vi "ArduinoMicro Module.vi"(5 "Enable":bool=TRUE, 6 "Timeout(s)":dbl=2.0, 7 "Command":T3, 8 "error in (no error)":errorcluster, 10 "VALVES":T1, 11 "VISA resource name":refnum<visa-resource-name>="COM39") -> (0 "error out":errorcluster, 1 "Output":T2, 2 "read string":string, 3 "TimeOut":bool, 4 "write string":string)   [LabVIEW 2017]
uses:
  ArduinoMicro Module Control.ctl
  KISSIA_VALVULAS.ctl
  <vilib>/Instr/_visa.llb/VISA Configure Serial Port (Instr).vi
panel:
  # "Input Data"
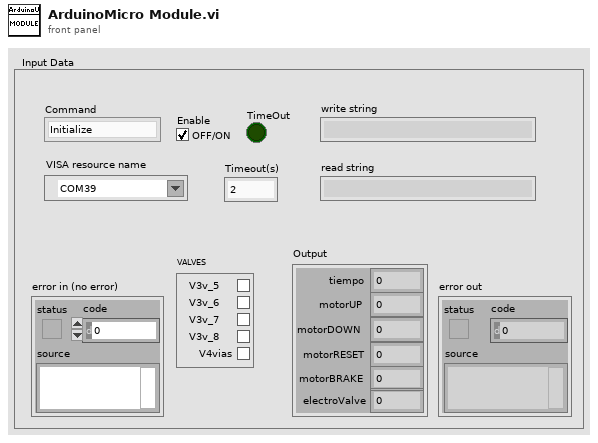
[diagram p1: front panel]
types:
  T1 = typedef "KISSIA_VALVULAS.ctl" = cluster{"V3v_5":bool, "V3v_6":bool, "V3v_7":bool, "V3v_8":bool, "V4vias":bool}
  T2 = cluster{"tiempo":dbl, "motorUP":dbl, "motorDOWN":dbl, "motorRESET":dbl, "motorBRAKE":dbl, "electroValve":dbl}
  T3 = typedef "ArduinoMicro Module Control.ctl" = enum16{"Initialize", "Read Data", "Write Data", "Enable", "Disable", "Shutdown"}
  T4 = cluster{"tiempo":dbl, "Valvula":dbl, "motorUP":dbl, "motorDOWN":dbl, "motorRESET":dbl, "motorBRAKE":dbl}
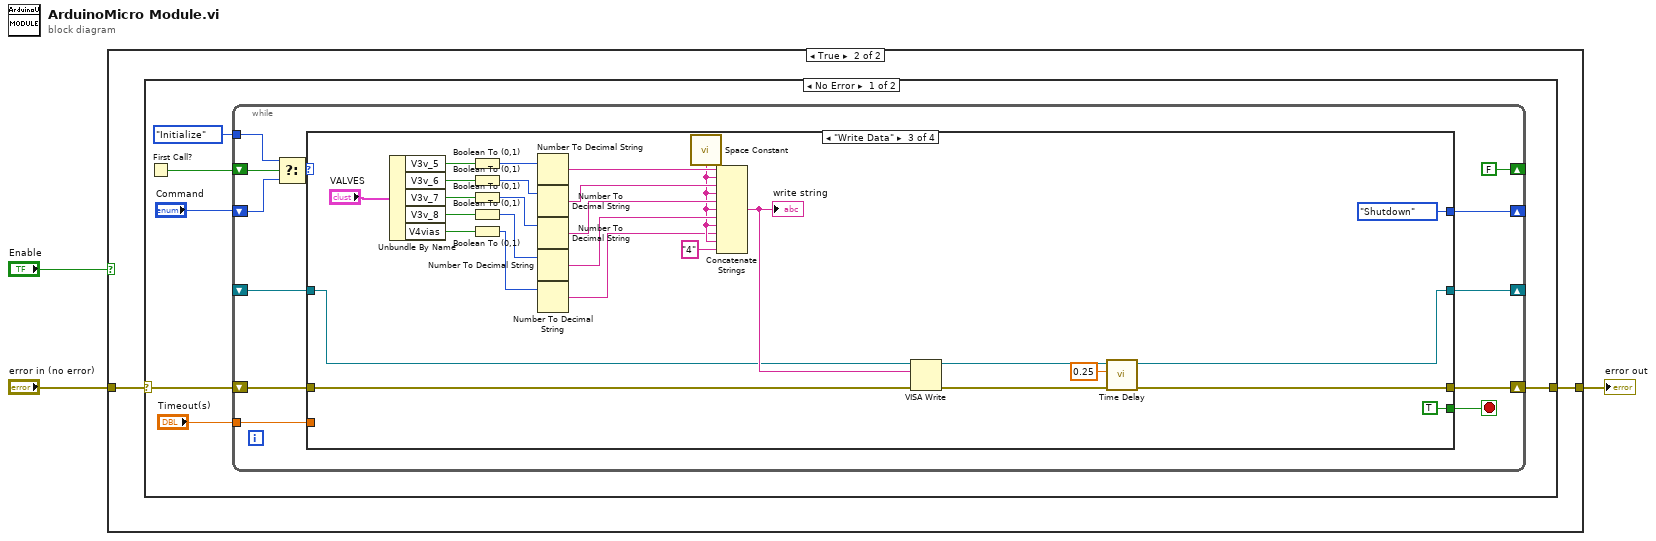
[diagram p0: block diagram]
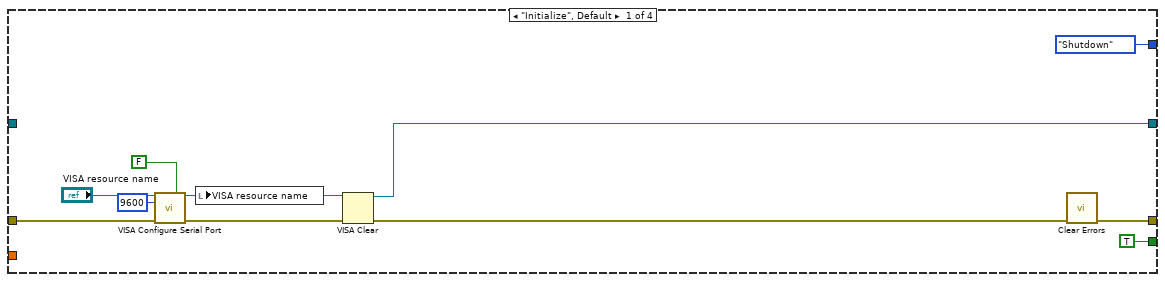
[diagram p3: hidden frame]
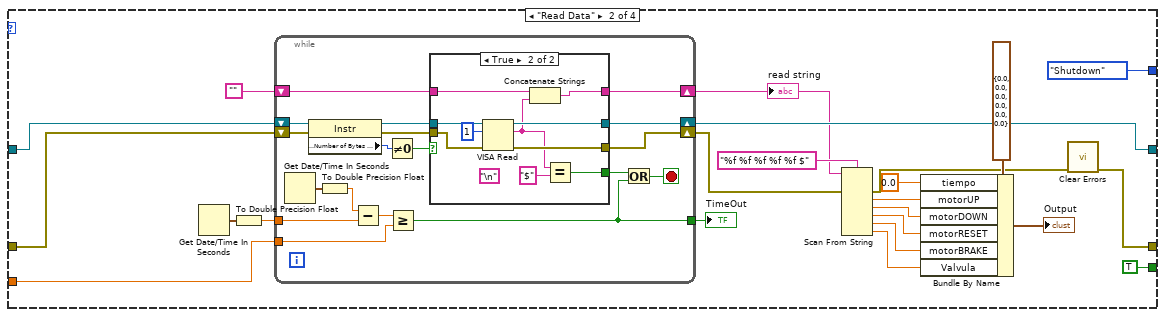
[diagram p4: hidden frame]
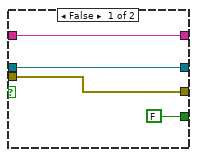
[diagram p5: hidden frame]
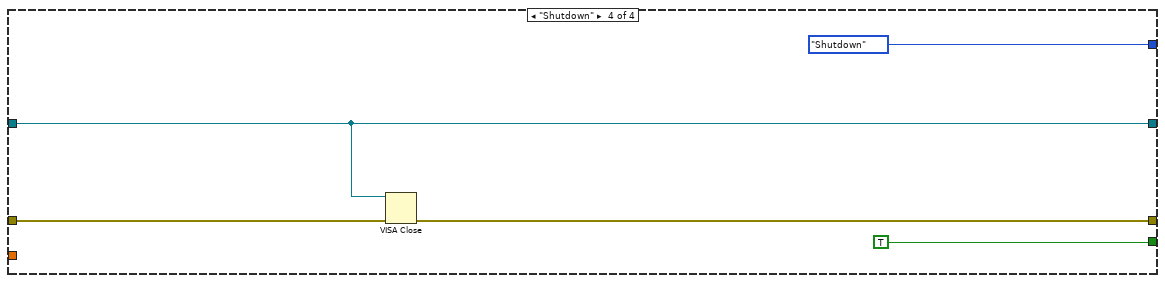
[diagram p6: hidden frame]
diagram:
  n1 = case shown="True" "Enable" {
    tunnel: "error in (no error)" -> [w4 w6]
    tunnel: [w4 w5] -> w2
    frame False {
    }
    frame True {
      n2 = case shown="No Error" w6 {
        selector: w6 -> [w10 w123]
        tunnel: [w9 w123] -> w5
        frame No Error {
          n3 = First Call?() -> (First Call?: T/F=w12:bool)
          n4 = while {
            shift-right: [w15] -> _
            shift-left: "Command" -> [w21]
            shift-right: [w18] -> w9
            shift-left: w10 -> [w19]
            shift-right: [FALSE ("First Call?: T/F")] -> _
            shift-left: w12 -> [w24]
            tunnel: ArduinoMicro_Module_Control."Initialize" ("t") -> [w23]
            shift-right: [w17] -> _
            shift-left: _ -> [w16]
            tunnel: "Timeout(s)" -> [w13]
            stop <- w14 stop-if-true
            n5 = Select(t=w23, s=w24, f=w21) -> (s? t:f=w20:T3)
            n6 = case shown="\"Write Data\"" w20 {
              tunnel: w19 -> [w30 w43 w91 w119]
              tunnel: [w27 w36 w93 w118] -> w18
              tunnel: [w25 w51 w115 w120] -> w17
              tunnel: w16 -> [_ w44 w92 w120]
              tunnel: [ArduinoMicro_Module_Control."Shutdown" ("t") ArduinoMicro_Module_Control."Shutdown" ("t") ArduinoMicro_Module_Control."Shutdown" ("t") ArduinoMicro_Module_Control."Shutdown" ("t")] -> w15
              tunnel: [TRUE ("Enable Termination\nChar (T)") TRUE ("Enable Termination\nChar (T)") TRUE ("Enable Termination\nChar (T)") TRUE ("Enable Termination\nChar (T)")] -> w14
              tunnel: w13 -> [_ w54 _ _]
              frame "Initialize", Default {
                n7 = call-poly "VISA Configure Serial Port"("VISA resource name"="VISA resource name", "Enable Termination\nChar (T)"=FALSE ("Enable Termination\nChar (T)"), "baud rate (9600)"=u32 9600, "error in (no error)"=w30) -> ("VISA resource name out"=w29:refnum<visa-resource-name>, "error out"=w28:errorcluster)  [unwired: 10 in]
                n8 = local write "VISA resource name"(w29) -> ()
                n9 = VISA Clear(VISA resource name=w29, error in (no error)=w28) -> (VISA resource name out=w25:refnum<visa-resource-name>, error out=w26:errorcluster)
                n10 = call <vilib>:"Clear Errors.vi"("error in (no error)"=w26) -> ("error out"=w27:errorcluster)  [unwired: 5 in, 1 out]
              }
              frame "Read Data" {
                n11 = Get Date/Time In Seconds() -> (seconds since 1Jan1904=w53:timestamp)
                n12 = To Double Precision Float(number=w53) -> (double precision float=w52:dbl)
                n13 = while {
                  tunnel: w52 -> [w73]
                  shift-right: [w69] -> w51
                  shift-left: w44 -> [w67]
                  shift-right: [w68] -> w38
                  shift-left: w43 -> [w66]
                  tunnel: w54 -> [w71]
                  tunnel: [w70] -> w55
                  shift-right: [w60] -> w47
                  shift-left: "" -> [w61]
                  stop <- w76 stop-if-true
                  n14 = Get Date/Time In Seconds() -> (seconds since 1Jan1904=w75:timestamp)
                  n15 = property class="Instr"(reference=w67, error in=w66) -> (reference out=w64:refnum<visa-resource-name>, error out=w65:errorcluster, "Serial Settings:Number of Bytes at Serial Port"=w63:u32)
                  n16 = To Double Precision Float(number=w75) -> (double precision float=w74:dbl)
                  n17 = Subtract(x=w74, y=w73) -> (x-y=w72:dbl)
                  n18 = Not Equal To 0?(x=w63) -> (x != 0?=w62:bool)
                  n19 = Greater Or Equal?(x=w72, y=w71) -> (x >= y?=w70:bool)
                  n20 = case shown="True" w62 {
                    tunnel: [w80 w90] -> w69
                    tunnel: [w79 w89] -> w68
                    tunnel: w65 -> [w79 w88]
                    tunnel: w64 -> [w80 w87]
                    tunnel: w61 -> [w78 w86]
                    tunnel: [w78 w85] -> w60
                    tunnel: [FALSE w82] -> w59
                    frame False {
                    }
                    frame True {
                      (unwired) "\n"
                      n21 = VISA Read(VISA resource name=w87, byte count=u32 1, error in (no error)=w88) -> (VISA resource name out=w90:refnum<visa-resource-name>, read buffer=w83:string, error out=w89:errorcluster)  [unwired: 1 out]
                      n22 = Concatenate Strings(w86, w83) -> (w85:string)
                      n23 = Equal?(x=w83, y="$" ("Mide")) -> (x = y?=w82:bool)
                    }
                  }
                  n24 = Or(x=w59, y=w70) -> (x .or. y?=w76:bool)
                }
                "read string" <- w47
                "TimeOut" <- w55
                n25 = Scan From String(format string="%f %f %f %f %f $", input string=w47, error in=w38) -> (error out=w37:errorcluster, output 1=w46:dbl, output 2=w45:dbl, output 3=w49:dbl, output 4=w40:dbl, output 5=w39:dbl)  [unwired: 6 in, 2 out]
                n26 = Bundle By Name(cluster=T4 {"tiempo"=0.0, "Valvula"=0.0, "motorUP"=0.0, "motorDOWN"=0.0, "motorRESET"=0.0, "motorBRAKE"=0.0} ("Output"), "tiempo"=0.0, "motorUP"=w46, "motorDOWN"=w45, "motorRESET"=w49, "motorBRAKE"=w40, "Valvula"=w39) -> (→"Output":T4)
                n27 = call <vilib>:"Clear Errors.vi"("error in (no error)"=w37) -> ("error out"=w36:errorcluster)  [unwired: 5 in, 1 out]
              }
              frame "Write Data" {
                n28 = Unbundle By Name("VALVES") -> ("V3v_5"=w113:bool, "V3v_6"=w112:bool, "V3v_7"=w111:bool, "V3v_8"=w110:bool, "V4vias"=w99:bool)
                n29 = Boolean To (0,1)(Boolean=w113) -> (0, 1=w109:i16)
                n30 = Boolean To (0,1)(Boolean=w112) -> (0, 1=w107:i16)
                n31 = Boolean To (0,1)(Boolean=w111) -> (0, 1=w106:i16)
                n32 = Boolean To (0,1)(Boolean=w110) -> (0, 1=w105:i16)
                n33 = Boolean To (0,1)(Boolean=w99) -> (0, 1=w98:i16)
                n34 = Number To Decimal String(number=w109) -> (decimal integer string=w108:string)  [unwired: 1 in]
                n35 = Number To Decimal String(number=w107) -> (decimal integer string=w104:string)  [unwired: 1 in]
                n36 = Number To Decimal String(number=w106) -> (decimal integer string=w103:string)  [unwired: 1 in]
                n37 = Number To Decimal String(number=w105) -> (decimal integer string=w102:string)  [unwired: 1 in]
                n38 = Number To Decimal String(number=w98) -> (decimal integer string=w95:string)  [unwired: 1 in]
                n39 = call <vilib>:"Space Constant.vi"() -> ("String"=w96:string)
                n40 = Concatenate Strings(w108, w96, w104, w96, w103, w96, w102, w96, w95, w96, "4" ("string")) -> (w101:string)
                "write string" <- w101
                n41 = VISA Write(VISA resource name=w92, write buffer=w101, error in (no error)=w91) -> (VISA resource name out=w115:refnum<visa-resource-name>, error out=w94:errorcluster)  [unwired: 1 out]
                n42 = call "Time Delay"("error in (no error)"=w94, "Delay Time (s)"=0.25) -> ("error out"=w93:errorcluster)  [unwired: 9 in]
              }
              frame "Shutdown" {
                n43 = VISA Close(VISA resource name=w120, error in (no error)=w119) -> (error out=w118:errorcluster)
              }
            }
          }
        }
        frame Error {
        }
      }
    }
  }
  "error out" <- w2
